vi "ASDA-A2_PR Event_Start.vi"(8 "error in":errorcluster, 11 "Buffer Data In":T1) -> (0 "error out":errorcluster, 3 "Buffer Data Out":T1)   [LabVIEW 2016]
uses:
  Data Def/ASDA-A2_Buffer Data.ctl
  Data Def/ASDA-A2_Write Register Data.ctl
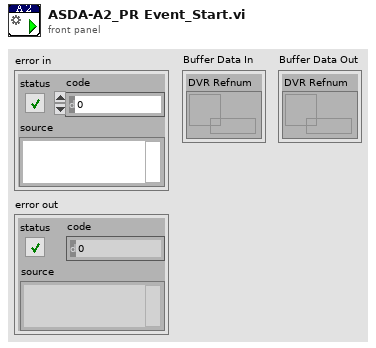
[diagram p1: front panel]
types:
  T1 = typedef "ASDA-A2_Buffer Data.ctl" = cluster{"DVR Refnum":refnum<data-value>}
  T2 = typedef "ASDA-A2_Write Register Data.ctl" = cluster{"Address":u16, "Max Value":u32, "Min Value":u32, "Value":u32, "Type":enum16{"16 Bits", "32 Bits"}, "Page":string, "Description":string}
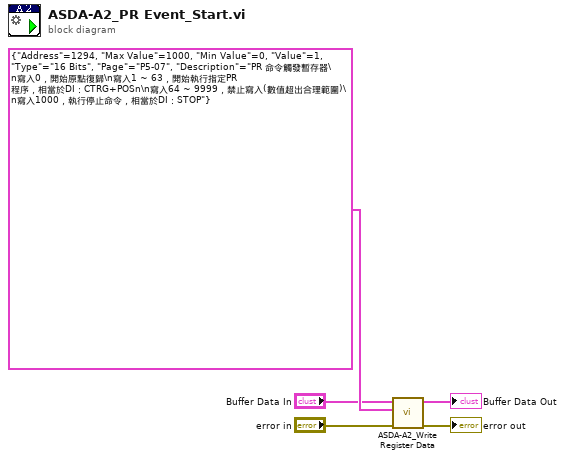
[diagram p0: block diagram]
diagram:
  n1 = call "ASDA-A2_Write Register Data.vi"("error in"="error in", "Write Register Data"=T2 {"Address"=1294, "Max Value"=1000, "Min Value"=0, "Value"=1, "Type"=enum."16 Bits", "Page"="P5-07", "Description"="PR 命令觸發暫存器\n寫入0，開始原點復歸\n寫入1 ~ 63，開始執行指定PR 程序，相當於DI：CTRG+POSn\n寫入64 ~ 9999，禁止寫入(數值超出合理範圍)\n寫入1000，執行停止命令，相當於DI：STOP"}, "Buffer Data In"="Buffer Data In") -> ("error out"=→"error out":errorcluster, "Buffer Data Out"=→"Buffer Data Out":T1)  [unwired: 7 in]
